vi "Subvi gated pixel clock.vi"(9 "Nmax lines":u16) -> ()   [LabVIEW 2017]
uses:
  <vilib>/Platform/TimedLoop/XDataNode/timing_clust.ctl
  <vilib>/Platform/TimedLoop/XDataNode/nitl_modes.ctl
  <vilib>/Platform/TimedLoop/XDataNode/wakeup.ctl
  <vilib>/rvi/Emulation/niFpgaSctlEmulationGetInTimedLoop.vi
  <vilib>/rvi/Emulation/niFpgaEmulationReportErrorSimple.vi
  <vilib>/rvi/Emulation/niFpgaGetClockAttributes.vi
  <vilib>/rvi/Emulation/niFpgaCriticalErrorInLSC.vi
  <vilib>/rvi/Emulation/niFpgaProcessEmulError.vi
  Detector/GV pixel clock.vi
  Detector/GV line clock change.vi
  <vilib>/Platform/TimedLoop/XDataNode/XDataNode.xnode
  Detector/GV gated pixel clock change.vi
  <vilib>/Platform/TimedLoop/XDataNode/XDNodeRunTimeDep.lvlib
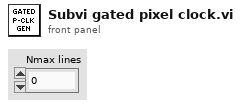
[diagram p1: front panel]
types:
  T1 = typedef "XDNodeRunTimeDep.lvlib/timing_clust.ctl" = cluster{"Expected End [f-1]":u64, "Actual End [f-1]":u64, "Finished Late? [f-1]":bool, "Expected End [i-1]":u64, "Actual End [i-1]":u64, "Finished Late? [i-1]":bool, "Expected Start [i]":u64, "Actual Start [i]":u64, "Expected Start [f]":u64, "Actual Start [f]":u64, "Source Name":string, "Structure Name":string, "Period":i64, "Deadline":i64, "Offset":i64, "Start":i64, "Priority":i32, "Timeout":i32, "Mode":T2, "Wakeup Reason":T3, "Error":errorcluster, "Source Type":string, "Secondary Source Type":string, "Global End Time":u64, "Global Start Time":u64, "Frame Duration":u64, "Iteration Duration":u64, "Assigned CPU":i32, "I/O Scan Engine Mode":u32}
  T2 = typedef "XDNodeRunTimeDep.lvlib/nitl_modes.ctl" = enum32{"No Change", "Process missed periods, maintain original phase", "Discard missed periods, maintain original phase", "Process missed periods, ignore original phase", "Discard missed periods, ignore original phase"}
  T3 = typedef "XDNodeRunTimeDep.lvlib/wakeup.ctl" = enum32{"Normal", "Aborted", "Asynchronous wakeup", "Timing source error", "Timed loop error", "Timeout"}
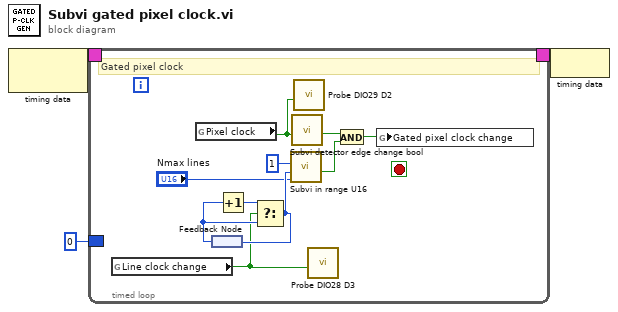
[diagram p0: block diagram]
diagram:
  n1 = node-c288() -> (w3:T1)  [unwired: 1 in]
  n2 = timed-loop {
    timing: w3 -> [_]
    timing-out: [_] -> w2
    border: u16 0 -> [_]
    stop <- _ stop-if-true
    # "Gated pixel clock"
    n3 = global read "GV line clock change.vi" "Line clock change"() -> (w4:bool)
    n4 = global read "GV pixel clock.vi" "Pixel clock"() -> (w6:bool)
    n5 = feedback #1() -> (w7:u16)
    n6 = Increment(x=w7) -> (x+1=w9:u16)
    n7 = Select(t=w9, s=w4, f=w7) -> (s? t:f=w10:u16)
    n8 = feedback-in #1(w10) -> ()
    n9 = call "Subvi in range U16.vi"("Max"="Nmax lines", "Input"=w10, "Min"=u16 1) -> ("In range"=w8:bool)  [unwired: 8 in]
    n10 = call "Subvi detector edge change bool.vi"("Input"=w6) -> ("Output"=w13:bool)  [unwired: 8 in]
    n11 = call "Probe DIO29 D2.vi"("D2"=w6) -> ()  [unwired: 11 in]
    n12 = call "Probe DIO28 D3.vi"("D3"=w4) -> ()  [unwired: 11 in]
    n13 = And(x=w13, y=w8) -> (x .and. y?=w12:bool)
    n14 = global write "GV gated pixel clock change.vi" "Gated pixel clock change"(w12) -> ()
  }
  n15 = node-c288(w2) -> ()
